vi "allNote.vi"(4 "起始音":T1={"音名"=enum."A", "度"=enum."0", "變音記號"=enum.""}, 6 "KeyNumber":i32=52) -> (2 "音名Array":string[](array[string]), 3 "Allnote":string[][](array[string]))   [LabVIEW 2015]
uses:
  Note.ctl
panel:
  out "重升":string[](array[string])
  out "ど":string[](array[string])
  out "重降":string[](array[string])
  out "降":string[](array[string])
  out "基本音":string[](array[string])
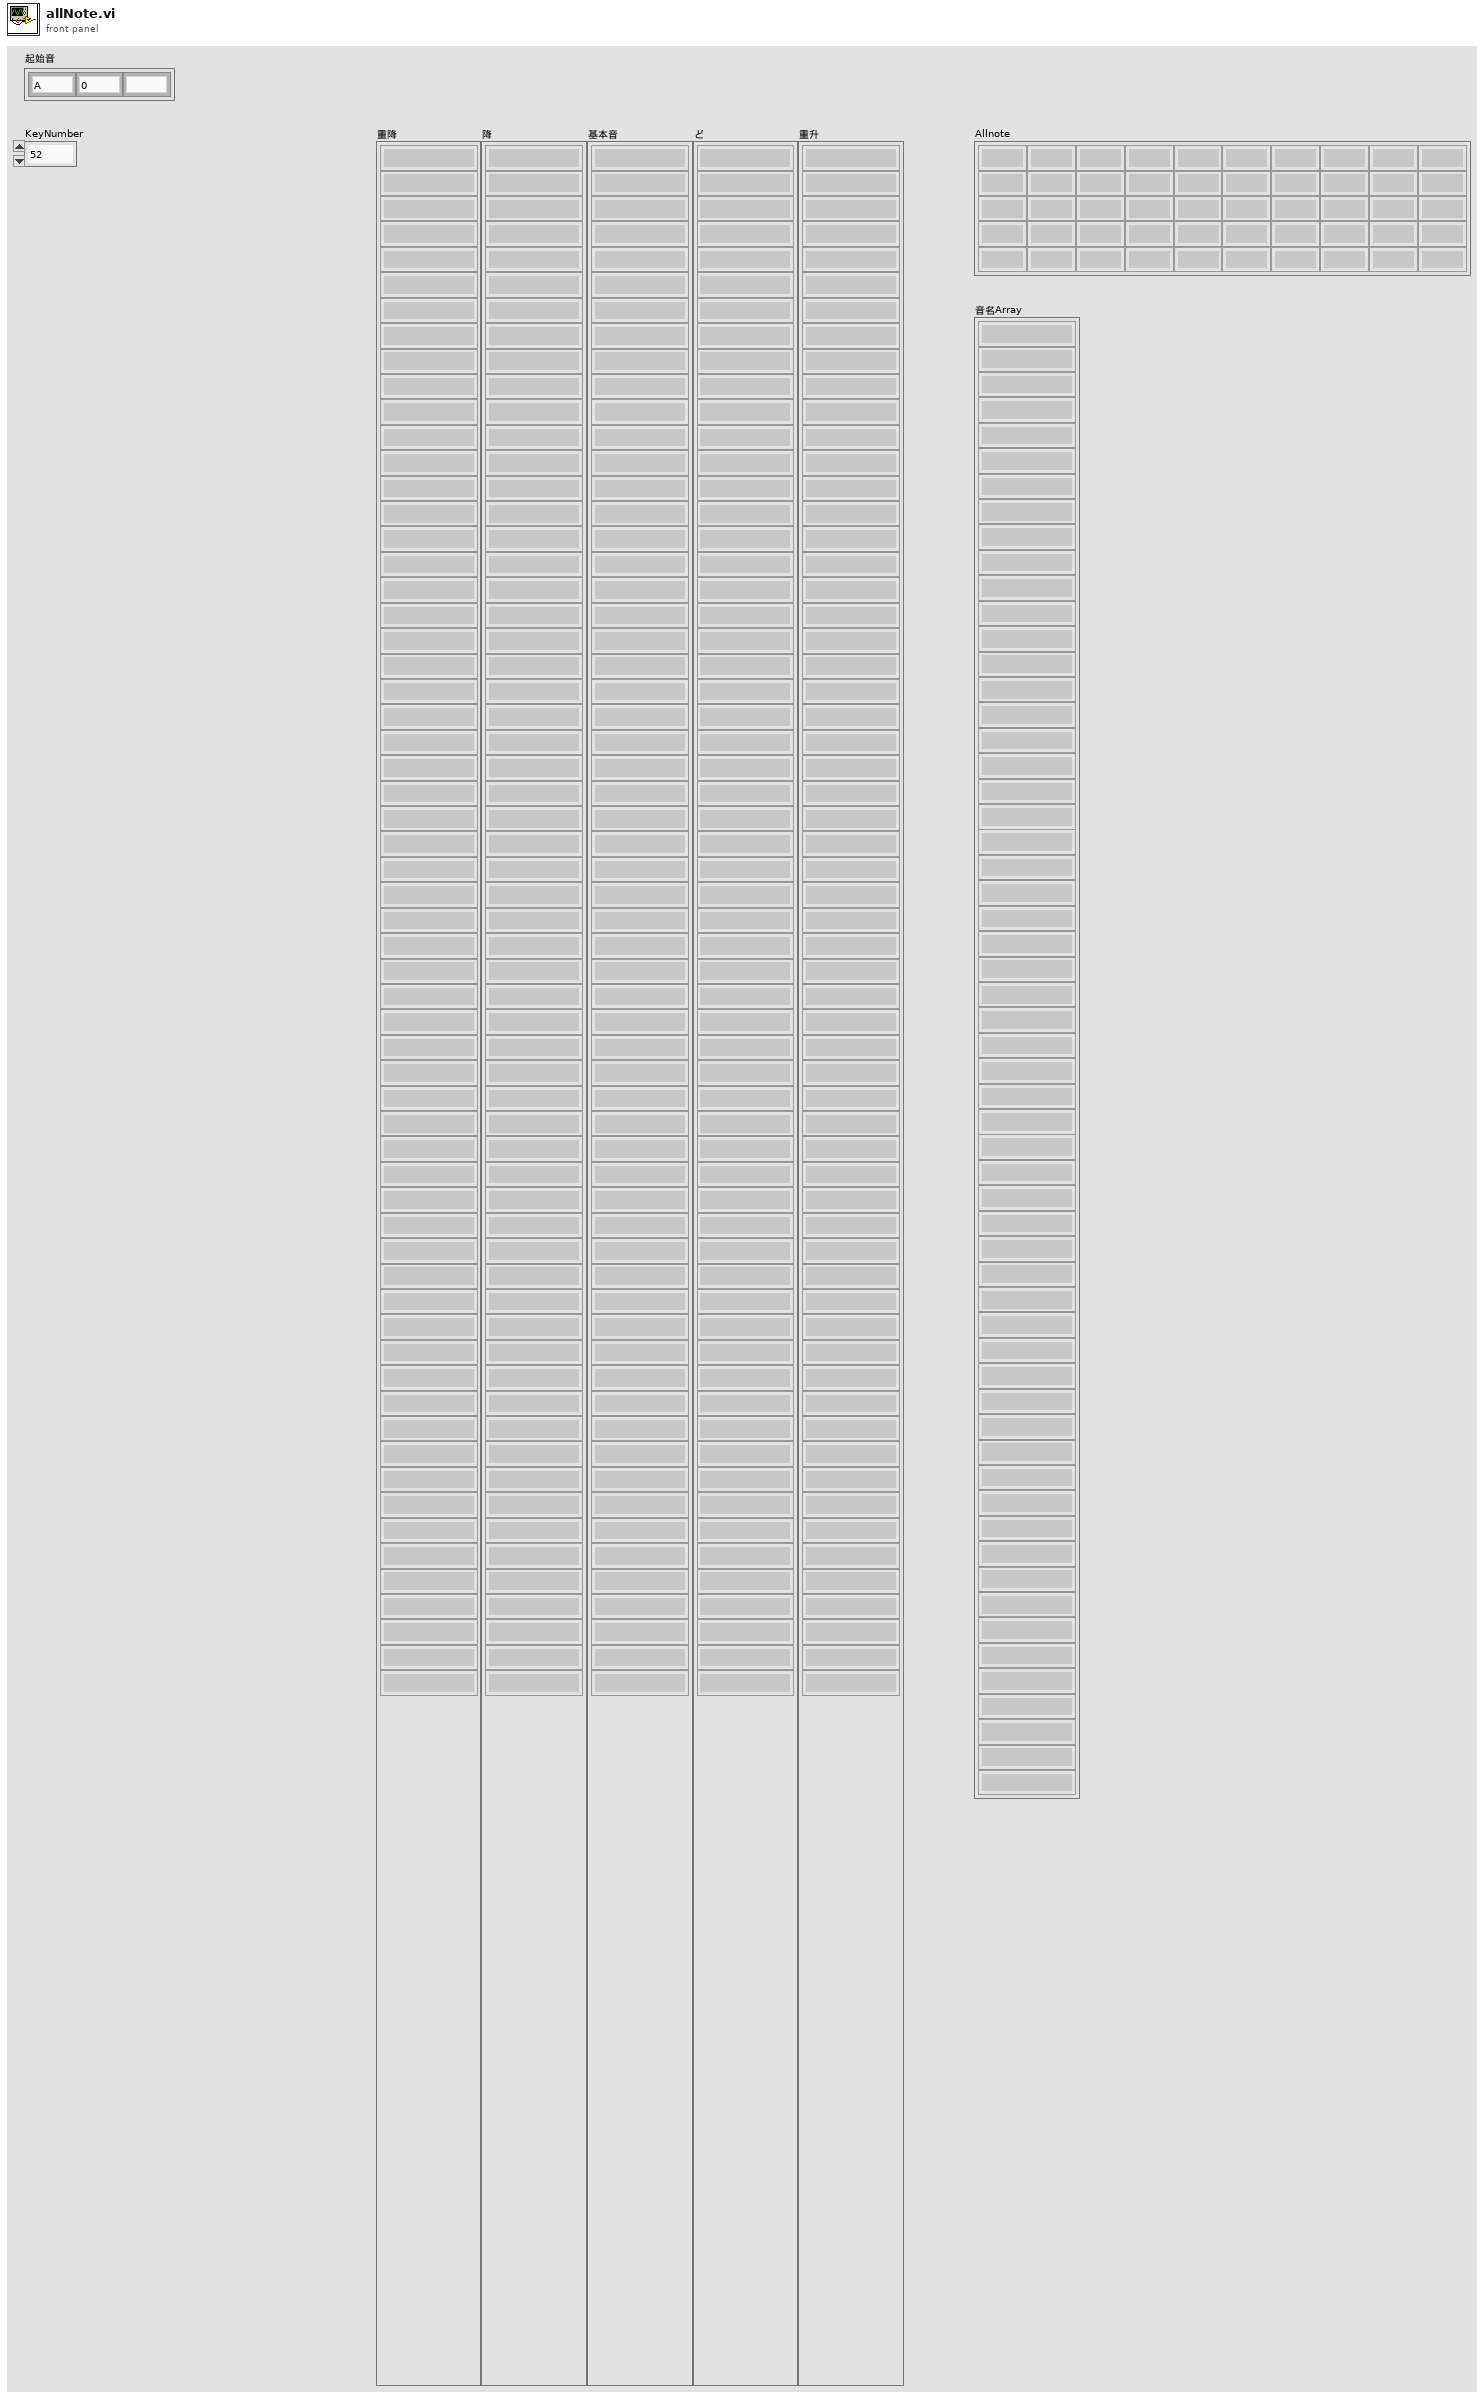
[diagram p1: front panel]
types:
  T1 = typedef "Note.ctl" = cluster{"音名":enum16{"C", "D", "E", "F", "G", "A", "B"}, "度":enum16{"0", "1", "2", "3", "4", "5", "6", "7", "8"}, "變音記號":enum16{"bb", "b", "", "#", "x"}}
  T2 = enum16{"0", "1", "2", "3", "4", "5", "6", "7", "8"}
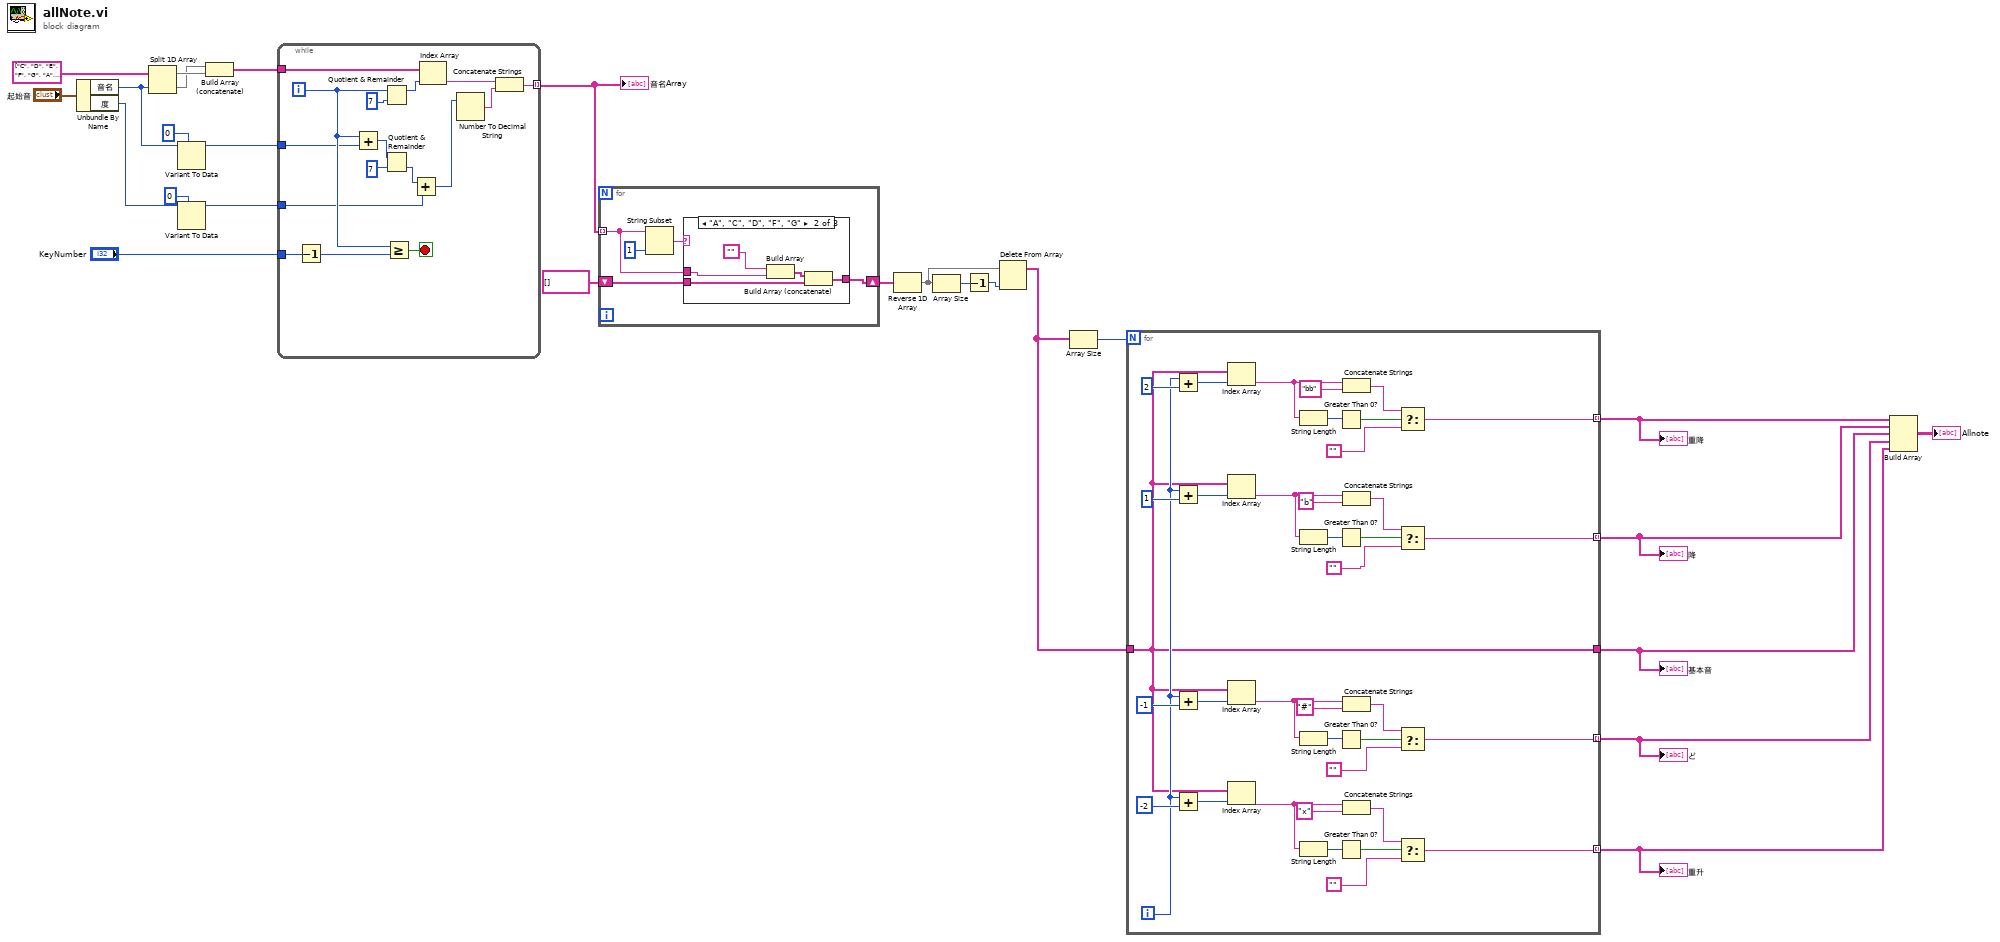
[diagram p0: block diagram]
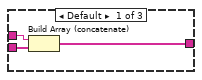
[diagram p2: hidden frame]
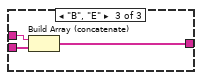
[diagram p3: hidden frame]
diagram:
  n1 = Unbundle By Name("起始音") -> ("音名"=w10:enum16{"C", "D", "E", "F", "G", "A", "B"}, "度"=w8:T2)
  n2 = Split 1D Array(array=string[] ["C", "D", "E", "F", "G", "A", "B"], index=w10) -> (first subarray=w16:string[], second subarray=w15:string[])
  n3 = Variant To Data(type=0 ("y"), Variant=w10) -> (data=w7:i32)  [unwired: 1 in, 1 out]
  n4 = Variant To Data(type=0 ("y"), Variant=w8) -> (data=w6:i32)  [unwired: 1 in, 1 out]
  n5 = Build Array (concatenate)(w15, w16) -> (w14:string[])
  n6 = while {
    tunnel: w14 -> [w40]
    tunnel: [w36] -> w21 mode=indexing
    tunnel: "KeyNumber" -> [w28]
    tunnel: w7 -> [w34]
    tunnel: w6 -> [w30]
    i -> [w35]
    stop <- w41 stop-if-true
    n7 = Decrement(x=w28) -> (x-1=w27:i32)
    n8 = Add(x=w35, y=w34) -> (x+y=w33:i32)
    n9 = Quotient & Remainder(x=w35, y=7) -> (x-y*floor(x/y)=w39:i32)  [unwired: 1 out]
    n10 = Quotient & Remainder(x=w33, y=7) -> (floor(x/y)=w31:i32)  [unwired: 1 out]
    n11 = Greater Or Equal?(x=w35, y=w27) -> (x >= y?=w41:bool)
    n12 = Add(x=w31, y=w30) -> (x+y=w29:i32)
    n13 = Index Array(array=w40, index=w39) -> (element=w38:string)
    n14 = Number To Decimal String(number=w29) -> (decimal integer string=w37:string)  [unwired: 1 in]
    n15 = Concatenate Strings(w38, w37) -> (w36:string)
  }
  "音名Array" <- w21
  n16 = for {
    tunnel: w21 -> [w45] mode=indexing
    shift-right: [w43] -> w25
    shift-left: string[] [] -> [w44]
    n17 = String Subset(string=w45, length (rest)=1 ("length (rest)")) -> (substring=w46:string)  [unwired: 1 in]
    n18 = case shown="\"A\", \"C\", \"D\", \"F\", \"G\"" w46 {
      tunnel: w45 -> [w50 w55 w58]
      tunnel: [w48 w52 w56] -> w43
      tunnel: w44 -> [w49 w53 w57]
      frame Default {
        n19 = Build Array (concatenate)(w50, w49) -> (w48:string[])
      }
      frame "A", "C", "D", "F", "G" {
        n20 = Build Array("", w55) -> (w54:string[])
        n21 = Build Array (concatenate)(w54, w53) -> (w52:string[])
      }
      frame "B", "E" {
        n22 = Build Array (concatenate)(w58, w57) -> (w56:string[])
      }
    }
  }
  n23 = Reverse 1D Array(array=w25) -> (reversed array=w24:string[])
  n24 = Array Size(array=w24) -> (size(s)=w23:i32)
  n25 = Decrement(x=w23) -> (x-1=w22:i32)
  n26 = Delete From Array(array=w24, index=w22) -> (array with subset deleted=w3:string[])  [unwired: 1 in, 1 out]
  n27 = Array Size(array=w3) -> (size(s)=w2:i32)
  n28 = for {
    N: w2 -> [_]
    tunnel: [w68] -> w20 mode=indexing
    tunnel: [w70] -> w12 mode=indexing
    tunnel: [w66] -> w19 mode=indexing
    tunnel: [w64] -> w18 mode=indexing
    tunnel: [w59] -> w4
    tunnel: w3 -> [w59]
    i -> [w86]
    n29 = Add(x=w86, y=2) -> (x+y=w92:i32)
    n30 = Add(x=w86, y=1) -> (x+y=w93:i32)
    n31 = Add(x=w86, y=-1) -> (x+y=w91:i32)
    n32 = Add(x=w86, y=-2) -> (x+y=w88:i32)
    n33 = Index Array(array=w59, index=w92) -> (element=w74:string)
    n34 = Index Array(array=w59, index=w93) -> (element=w75:string)
    n35 = Index Array(array=w59, index=w91) -> (element=w73:string)
    n36 = Index Array(array=w59, index=w88) -> (element=w72:string)
    n37 = String Length(string=w74) -> (length=w80:i32)
    n38 = String Length(string=w75) -> (length=w83:i32)
    n39 = String Length(string=w73) -> (length=w79:i32)
    n40 = String Length(string=w72) -> (length=w76:i32)
    n41 = Greater Than 0?(x=w80) -> (x > 0?=w81:bool)
    n42 = Greater Than 0?(x=w83) -> (x > 0?=w82:bool)
    n43 = Greater Than 0?(x=w79) -> (x > 0?=w78:bool)
    n44 = Greater Than 0?(x=w76) -> (x > 0?=w77:bool)
    n45 = Concatenate Strings(w74, "bb" ("string")) -> (w71:string)
    n46 = Concatenate Strings(w75, "b" ("string")) -> (w69:string)
    n47 = Concatenate Strings(w73, "#" ("string")) -> (w67:string)
    n48 = Concatenate Strings(w72, "x" ("string")) -> (w65:string)
    n49 = Select(t=w71, s=w81, f="") -> (s? t:f=w70:string)
    n50 = Select(t=w69, s=w82, f="") -> (s? t:f=w68:string)
    n51 = Select(t=w67, s=w78, f="") -> (s? t:f=w66:string)
    n52 = Select(t=w65, s=w77, f="") -> (s? t:f=w64:string)
  }
  "基本音" <- w4
  "降" <- w20
  "重降" <- w12
  "ど" <- w19
  "重升" <- w18
  n53 = Build Array(w12, w20, w4, w19, w18) -> (→"Allnote":string[][])
